vi "Convert 1DDbl to DDT 2.vi"(2 "Array":dbl[](array[numeric]) format="%0.2f") -> (4 "Dynamic Data Type":dynamicdata(graph))   [LabVIEW 2018]
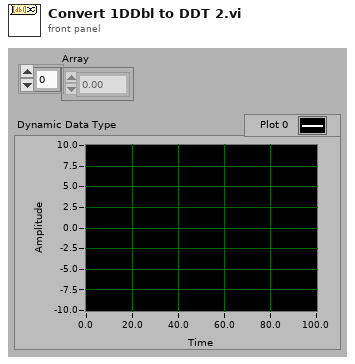
[diagram p1: front panel]
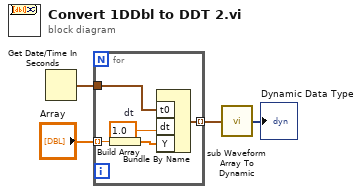
[diagram p0: block diagram]
diagram:
  n1 = Get Date/Time In Seconds() -> (seconds since 1Jan1904=w1:timestamp)
  n2 = for {
    tunnel: "Array" -> [w9] mode=indexing
    tunnel: [w7] -> w3 mode=indexing
    tunnel: w1 -> [w5]
    w6 = 1.0  # dt
    n3 = Build Array(w9) -> (w8:dbl[])
    n4 = Bundle By Name("t0"=w5, "dt"=w6, "Y"=w8) -> (w7:waveform(dbl))  [unwired: 1 out]
  }
  n5 = call "sub Waveform Array To Dynamic.vi"("Input"=w3) -> ("Output"=→"Dynamic Data Type":dynamicdata)  [unwired: 4 out]
